vi "usb write bit File init.vi"(11 "blkCnt_512B":i32) -> ()   [LabVIEW 2018, in "Dll1_x64_191014_0.lvlib"]
doc: "__declspec(dllexport) void usb_write_bitFile_init(int blkCnt_512B);"
uses:
  Dll1_x64_191014_0.lvlib
  Dll1.dll
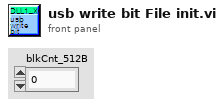
[diagram p1: front panel]
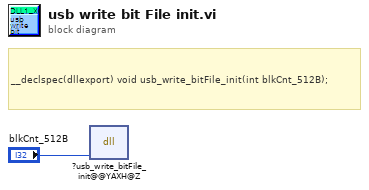
[diagram p0: block diagram]
diagram:
  # "__declspec(dllexport) void usb_write_bitFile_init(int blkCnt_512B);"
  n1 = dll-call lib="PTH2zabs CUsersLenovoDesktopDHCC실험2#lux image capture_0.9.1.1_Temporaryuser.libDll1_x64_191014_0Dll1.*" fn="?usb_write_bitFile_init@@YAXH@Z"("blkCnt_512B"="blkCnt_512B") -> ()  [unwired: 5 in, 2 out]
